vi "SubSystems.vi"(8 "error in":errorcluster) -> ()   [LabVIEW 2017]
doc: "This VI calls the various robot subsystems that will then run in parallel. New subSystems will automatlically script code to make the call."
uses:
  <vilib>/Rock Robotics/WPI/ThirdParty/Sensors/navX/_Processing Loop/FRIC_navX_Internal_I2C_ProcessingLoop.vi
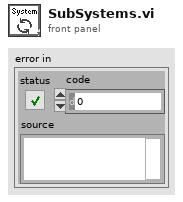
[diagram p1: front panel]
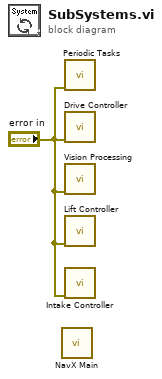
[diagram p0: block diagram]
diagram:
  n1 = call-poly <vilib>:"NavX Main.vi"() -> ()  [unwired: 12 in]
  n2 = call "Periodic Tasks.vi"("error in"="error in") -> ()  [unwired: 1 in, 10 out]
  n3 = call "Drive Controller.vi"("error in"="error in") -> ()  [unwired: 11 in]
  n4 = call "Vision Processing.vi"("error in (no error)"="error in") -> ()  [unwired: 7 in]
  n5 = call "Lift Controller.vi"("error in"="error in") -> ()  [unwired: 11 in]
  n6 = call "Intake Controller.vi"("error in"="error in") -> ()  [unwired: 11 in]
